vi "Configure and Start Acoustic AI.vi"(8 "error in":errorcluster, 11 "PAS in":refnum<class "PAS.lvclass">) -> (0 "error out":errorcluster, 3 "PAS out":refnum<class "PAS.lvclass">)   [LabVIEW 2014, in "PAS.lvclass"]
doc: "Configure and start the high frequency task for collecting the data microphone and/or photodiode data. The default VI starts a task named PAS Laser AI and stuffs it into the variable <b>acoustic</b>."
uses:
  PAS.lvclass
  PAS.lvclass/PAS.ctl
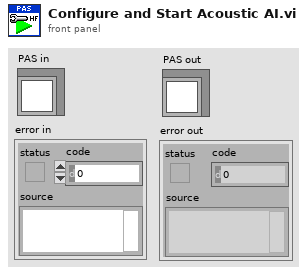
[diagram p1: front panel]
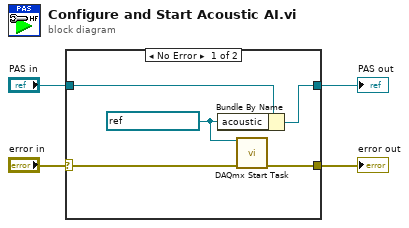
[diagram p0: block diagram]
diagram:
  n1 = case shown="No Error" "error in" {
    selector: "error in" -> [w6 w11]
    tunnel: [w5 w11] -> w3
    tunnel: [w8 w10] -> w1
    tunnel: "PAS in" -> [w9 w10]
    frame No Error {
      w7 = refnum<k21> "PAS Laser AI" ("DAQmxTasks.acoustic")
      n2 = Bundle By Name(cluster=w9, "acoustic"=w7) -> (w8:refnum<class "PAS.lvclass">)
      n3 = call <vilib>:"DAQmx Start Task.vi"("task/channels in"=w7, "error in"=w6) -> ("error out"=w5:errorcluster)  [unwired: 12 in, 1 out]
    }
    frame Error {
    }
  }
  "error out" <- w3
  "PAS out" <- w1
